vi "fb_microstep.vi"(1 "Sensor":enum16{"l", "r", "both"}(ring), 3 "precision":dbl, 4 "R_Taget_Zeta":i32, 5 "taget_IR_L":dbl, 6 "L_Taget_Zeta":i32, 7 "taget_IR_R":dbl, 8 "SamplingNUM":i32, 9 "Step":i32, 10 "Delay":i32, 11 "Stop Mode":string(combo)) -> (0 "Done":bool)   [LabVIEW 2017]
uses:
  <vilib>/myRIO/Instrument Drivers/Onboard IO/AI/typedefs/AI Reference.ctl
  <vilib>/myRIO/Common/Instrument Driver Framework/Utilities/typedefs/myRIO Generic Hardware Reference.ctl
  <vilib>/myRIO/Common/Instrument Driver Framework/Utilities/typedefs/Hardware Version Enum.ctl
  <vilib>/myRIO/Common/Instrument Driver Framework/Utilities/typedefs/myRIO v1.0 Reference.ctl
  <vilib>/myRIO/Common/Instrument Driver Framework/Utilities/typedefs/Generic FPGA Reference.ctl
  <vilib>/myRIO/Common/Instrument Driver Framework/myRIO v1.0/AI/typedefs/AI Channels List.ctl
  <vilib>/myRIO/Common/Instrument Driver Framework/myRIO v1.0/AI/typedefs/AI Channels Enum.ctl
  <vilib>/myRIO/Common/Instrument Driver Framework/Utilities/typedefs/Analog Scaling Constants List.ctl
  <vilib>/myRIO/Common/Instrument Driver Framework/Utilities/typedefs/Analog Scaling Constants.ctl
  <vilib>/userdefined/High Color/nirio_resource_hc.ctl
  <vilib>/myRIO/Common/Instrument Driver Framework/Utilities/vis/Is FPGA Ref Available.vi
  <vilib>/myRIO/Common/Instrument Driver Framework/myRIO v1.0/AI/vis/myRIO v1.1 Open AI.vi
  <vilib>/myRIO/Instrument Drivers/Onboard IO/AI/vis/Read.vi
  <vilib>/Analysis/baseanly.llb/Mean (DBL).vi
  <vilib>/myRIO/Common/Instrument Driver Framework/Utilities/vis/Validate Channels.vi
  <vilib>/myRIO/Common/Instrument Driver Framework/myRIO v1.0/AI/vis/myRIO v1.0 Reserve AI.vi
  <vilib>/myRIO/Common/Instrument Driver Framework/myRIO v1.0/AI/vis/myRIO v1.0 Build MUX Configuration AI.vi
  <vilib>/myRIO/Common/Instrument Driver Framework/myRIO v1.0/Resource Manager/vis/myRIO v1.0 Reserve Channel List.vi
  <vilib>/myRIO/Common/Instrument Driver Framework/myRIO v1.0/Resource Manager/vis/myRIO v1.0 Reserve Channel.vi
  <vilib>/myRIO/Common/Instrument Driver Framework/myRIO v1.0/Resource Manager/vis/myRIO v1.0 Unreserve Channel.vi
  <vilib>/myRIO/Common/Instrument Driver Framework/myRIO v1.0/Resource Manager/vis/myRIO v1.0 Build Mutex Name.vi
  <vilib>/Utility/VariantDataType/GetNumericInfo.vi
  <vilib>/Utility/error.llb/Error Cluster From Error Code.vi
  <vilib>/myRIO/Common/Instrument Driver Framework/myRIO v1.0/myRIO v1.1 Open.vi
  <vilib>/myRIO/Common/Instrument Driver Framework/myRIO v1.0/AI/vis/myRIO v1.0 Get Scaling Constants AI.vi
  <vilib>/myRIO/Common/Instrument Driver Framework/Utilities/vis/IO Manager.vi
  <vilib>/myRIO/Common/Instrument Driver Framework/Utilities/vis/Configuration Manager.vi
  <vilib>/myRIO/Common/Instrument Driver Framework/myRIO v1.0/myRIO v1.0 Close.vi
  <vilib>/myRIO/Common/Instrument Driver Framework/myRIO v1.0/AI/vis/myRIO v1.0 Read AI.vi
  Constant.vi
  <vilib>/myRIO/Express VI/Onboard IO/AI/AI Express VI.xnode
  <vilib>/myRIO/Instrument Drivers/Onboard IO/AI/vis/myRIO AI Open.xnode
  <vilib>/myRIO/Instrument Drivers/Onboard IO/AI/AI.lvlib
  <vilib>/Analysis/NI_AALBase.lvlib
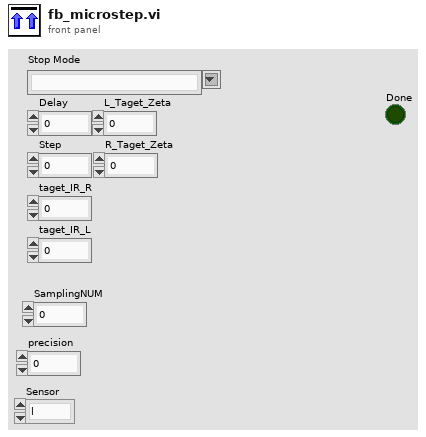
[diagram p1: front panel]
types:
  T1 = typedef "AI.lvlib/AI Reference.ctl" = cluster{"myRIO Reference":T2, "AI Channels List":T6, "AI Scaling Constants List":T8}
  T2 = typedef "myRIO Generic Hardware Reference.ctl" = cluster{"myRIO Model":T3, "myRIO Hardware Reference":T4}
  T3 = typedef "Hardware Version Enum.ctl" = enum16{"Unknown", "myRIO-1900", "myRIO-1950", "roboRIO", "NI ELVIS RIO CM"}
  T4 = typedef "myRIO v1.0 Reference.ctl" = cluster{"Generic FPGA Reference":T5, "Allow multiple opens":bool}
  T5 = typedef "Generic FPGA Reference.ctl" = refnum<k20>
  T6 = typedef "AI Channels List.ctl" = T7[]
  T7 = typedef "AI Channels Enum.ctl" = enum16{"Not Connected", "AudioIn/Left", "AudioIn/Right", "C/AI0", "C/AI1", "A/AI0", "A/AI1", "A/AI2", "A/AI3", "B/AI0", "B/AI1", "B/AI2", "B/AI3", "AI/AI0", "AI/AI1", "AI/AI2", "AI/AI3"}
  T8 = typedef "Analog Scaling Constants List.ctl" = T9[]
  T9 = typedef "Analog Scaling Constants.ctl" = cluster{"LSB Weight (Volts)":dbl, "Offset (Volts)":dbl, "Signed?":bool}
  T10 = typedef "nirio_resource_hc.ctl" = tag
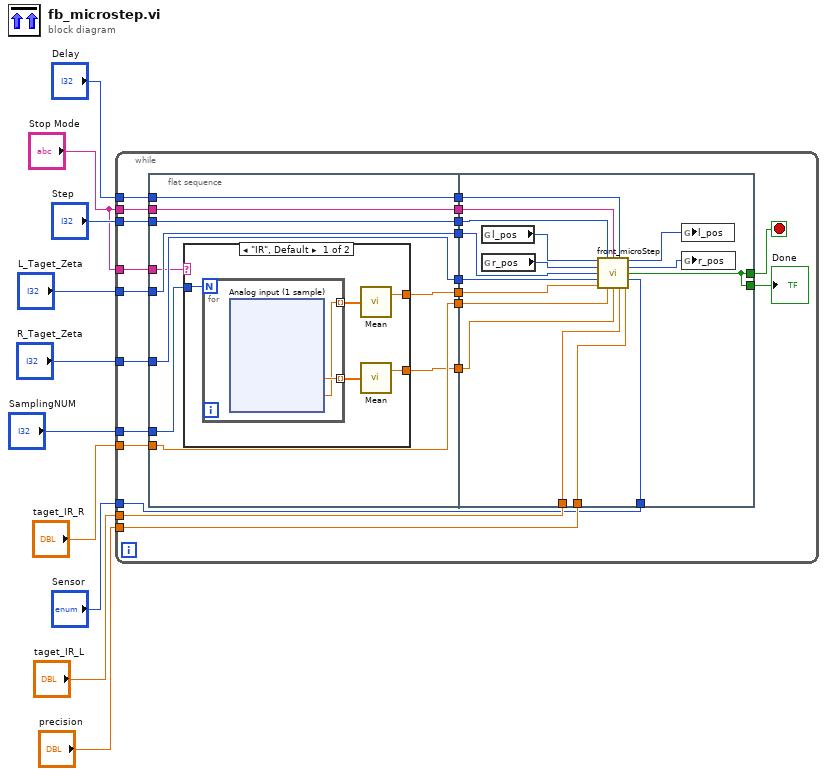
[diagram p0: block diagram]
diagram:
  n1 = while {
    tunnel: "Stop Mode" -> [w30]
    tunnel: "Delay" -> [w29]
    tunnel: "Step" -> [w28]
    tunnel: "L_Taget_Zeta" -> [w27]
    tunnel: "R_Taget_Zeta" -> [w26]
    tunnel: "taget_IR_R" -> [w25]
    tunnel: "SamplingNUM" -> [w18]
    tunnel: "taget_IR_L" -> [w15]
    tunnel: "precision" -> [w13]
    tunnel: "Sensor" -> [w12]
    tunnel: "Stop Mode" -> [w11]
    stop <- w31 stop-if-true
    n2 = flat-sequence {
      tunnel: w25 -> [w37]
      tunnel: w26 -> [w38]
      tunnel: w27 -> [w39]
      tunnel: w28 -> [w40]
      tunnel: w29 -> [w41]
      tunnel: w30 -> [w33]
      tunnel: [w33] -> w24
      tunnel: [w41] -> w23
      tunnel: [w40] -> w22
      tunnel: [w39] -> w21
      tunnel: [w38] -> w20
      tunnel: [w37] -> w19
      tunnel: w18 -> [w36]
      tunnel: [w35] -> w17
      tunnel: [w34] -> w16
      tunnel: w11 -> [w32]
      tunnel: [w89] -> w31
      tunnel: w24 -> [w98]
      tunnel: w23 -> [w97]
      tunnel: w22 -> [w96]
      tunnel: w21 -> [w95]
      tunnel: w20 -> [w94]
      tunnel: w19 -> [w93]
      tunnel: w17 -> [w92]
      tunnel: w16 -> [w91]
      tunnel: w15 -> [w90]
      tunnel: [w89] -> w14
      tunnel: w13 -> [w88]
      tunnel: w12 -> [w87]
      frame #0 {
        n3 = case shown="\"IR\", Default" w32 {
          tunnel: w36 -> [w46 _]
          tunnel: [w43 _] -> w35
          tunnel: [w42 _] -> w34
          frame "IR", Default {
            n4 = for {
              N: w46 -> [_]
              tunnel: [w48] -> w45 mode=indexing
              tunnel: [w47] -> w44 mode=indexing
              n5 = xnode "Analog input (1 sample)"() -> ("IR_L (A/AI0 (Pin 3))"=w48:dbl, "IR_R (A/AI1 (Pin 5))"=w47:dbl)  [unwired: 1 in, 1 out]
            }
            n6 = call-poly <vilib>:"Mean.vi"("X"=w44) -> ("mean"=w43:dbl)  [unwired: 1 out]
            n7 = call-poly <vilib>:"Mean.vi"("X"=w45) -> ("mean"=w42:dbl)  [unwired: 1 out]
          }
          frame "Zeta" {
          }
        }
      }
      frame #1 {
        n8 = global read "Constant.vi" "l_pos"() -> (w102:i32)
        n9 = global read "Constant.vi" "r_pos"() -> (w101:i32)
        n10 = call "front_microStep.vi"("Zeta_l"=w102, "Step"=w96, "Stop Mode"=w98, "Delay"=w97, "Zeta_R"=w101, "L_Taget_Zeta"=w95, "R_Taget_Zeta"=w94, "Sensor"=w87, "IR_R"=w92, "taget_IR_R"=w93, "IR_L"=w91, "taget_IR_L"=w90, "precision"=w88) -> ("OZeta_l"=w100:i32, "Ozeta_r"=w99:i32, "Done"=w89:bool)
        n11 = global write "Constant.vi" "l_pos"(w100) -> ()
        n12 = global write "Constant.vi" "r_pos"(w99) -> ()
      }
    }
    "Done" <- w14
  }
